vi "Get Scaling Factor.vi"(8 "error in (no error)":errorcluster, 11 "WeChat QR Code Detector in":refnum<class "WeChat QR Code Detector.lvclass">) -> (0 "error out":errorcluster, 2 "Scale Factor":sgl, 3 "WeChat QR Code Detector":refnum<class "WeChat QR Code Detector.lvclass">)   [LabVIEW 2020, in "feature_detection.lvlib" / "WeChat QR Code Detector.lvclass"]
doc: "Get the scaling factor to apply to the image before processing. This will be a value between 0 and 1.\n\nA value of -1 means to automatically set the scaling factor to give an image area of 160000 pixels."
uses:
  WeChat QR Code Detector.lvclass
  WeChat QR Code Detector.lvclass/WeChat QR Code Detector.ctl
  <vilib>/Utility/error.llb/Error Cluster From Error Code.vi
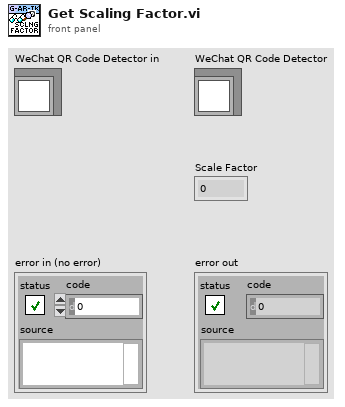
[diagram p1: front panel]
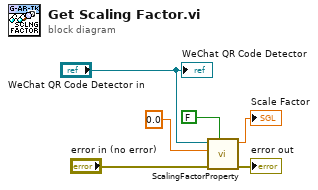
[diagram p0: block diagram]
diagram:
  n1 = call "ScalingFactorProperty.vi"("Write?"=FALSE, "error in (no error)"="error in (no error)", "Value in"=0.0 ("Value"), "QR Code Detector in"="WeChat QR Code Detector in") -> ("error out"=→"error out":errorcluster, "Value out"=→"Scale Factor":sgl)  [unwired: 6 in]
  "WeChat QR Code Detector" <- "WeChat QR Code Detector in"
